vi "GUI Remove PS.vi"(9 "PS Graph Selector":T2[](array[typedef]), 10 "Inverse PS Matrix Mapping":u32[][](array[numeric]), 11 "Actuation Network in":T1) -> (3 "Actuation Network out":T1)   [LabVIEW 2011, in "User Interface VIs.lvlib"]
uses:
  Types Definitions/Type BPM or PS Selector.ctl
  Types Definitions/Type Actuation Network Configuration.ctl
  User Interface VIs.lvlib
  Type Definitions.lvlib
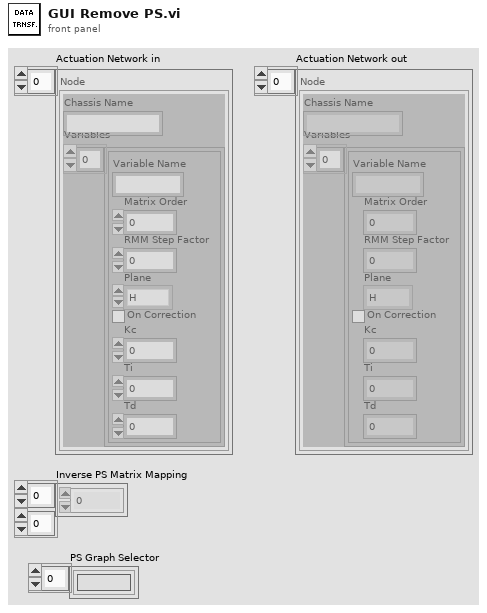
[diagram p1: front panel]
types:
  T1 = typedef "Type Definitions.lvlib/Type Actuation Network Configuration.ctl" = cluster{"Chassis Name":string, "Variables":cluster{"Variable Name":string, "Matrix Order":u32, "RMM Step Factor":dbl, "Plane":enum8{"H", "V"}, "On Correction":bool, "Kc":dbl, "Ti":dbl, "Td":dbl}[]}[]
  T2 = typedef "Type Definitions.lvlib/Type BPM or PS Selector.ctl" = cluster{"Name":string, "Active":bool}
  T3 = cluster{"Chassis Name":string, "Variables":cluster{"Variable Name":string, "Matrix Order":u32, "RMM Step Factor":dbl, "Plane":enum8{"H", "V"}, "On Correction":bool, "Kc":dbl, "Ti":dbl, "Td":dbl}[]}
  T4 = cluster{"Variable Name":string, "Matrix Order":u32, "RMM Step Factor":dbl, "Plane":enum8{"H", "V"}, "On Correction":bool, "Kc":dbl, "Ti":dbl, "Td":dbl}[]
  T5 = cluster{"Variable Name":string, "Matrix Order":u32, "RMM Step Factor":dbl, "Plane":enum8{"H", "V"}, "On Correction":bool, "Kc":dbl, "Ti":dbl, "Td":dbl}
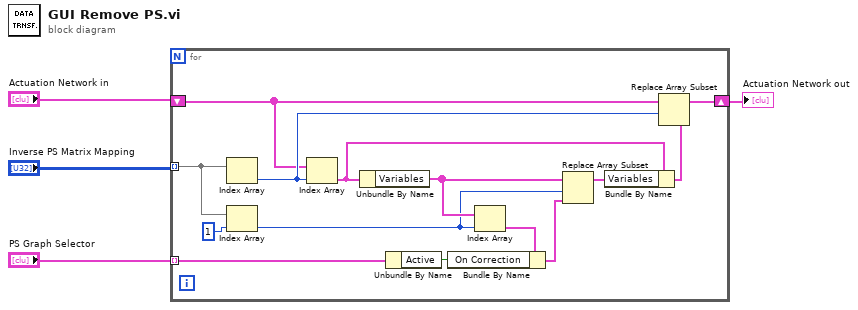
[diagram p0: block diagram]
diagram:
  n1 = for {
    tunnel: "Inverse PS Matrix Mapping" -> [w18] mode=indexing
    shift-right: [w9] -> w1
    shift-left: "Actuation Network in" -> [w5]
    tunnel: "PS Graph Selector" -> [w7] mode=indexing
    n2 = Index Array(array=w18) -> (element=w12:u32)  [unwired: 1 in]
    n3 = Index Array(array=w18, index=1) -> (element=w14:u32)
    n4 = Index Array(array=w5, index=w12) -> (element=w6:T3)
    n5 = Unbundle By Name(w6) -> ("Variables"=w15:T4)
    n6 = Unbundle By Name(w7) -> ("Active"=w16:bool)
    n7 = Index Array(array=w15, index=w14) -> (element=w17:T5)
    n8 = Bundle By Name(cluster=w17, "On Correction"=w16) -> (w13:T5)
    n9 = Replace Array Subset(array=w15, new element=w13, index=w14) -> (w11:T4)
    n10 = Bundle By Name(cluster=w6, "Variables"=w11) -> (w10:T3)
    n11 = Replace Array Subset(array=w5, new element=w10, index=w12) -> (w9:T1)
  }
  "Actuation Network out" <- w1
